vi "FP_Size to Largest Decoration.vi"(6 "Border Spacing (2 Px)":i32=2, 7 "Decoration index":i32, 8 "Error":errorcluster, 11 "VI Ref":refnum<vi>) -> (0 "Error Out":errorcluster, 2 "Front Panel.PanelBounds Out":T1, 3 "VI Ref Out":refnum<vi>)   [LabVIEW 2020]
doc: "Fits the vi's window to to the input GObject or largest decoration on the front panel"
uses:
  <vilib>/Utility/miscctls.llb/LVRectTypeDef.ctl
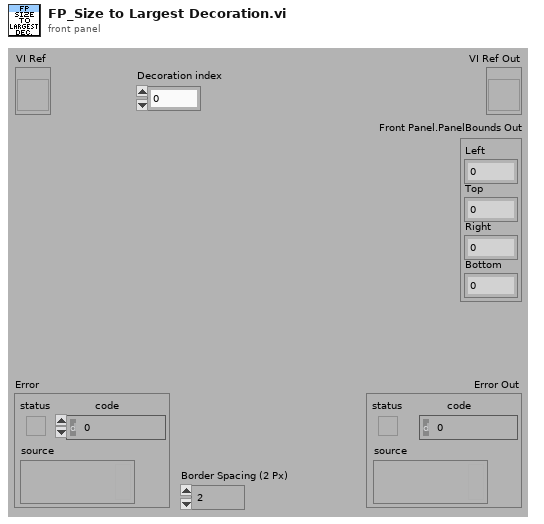
[diagram p1: front panel]
types:
  T1 = typedef "LVRectTypeDef.ctl" = cluster{"Left":i16, "Top":i16, "Right":i16, "Bottom":i16}
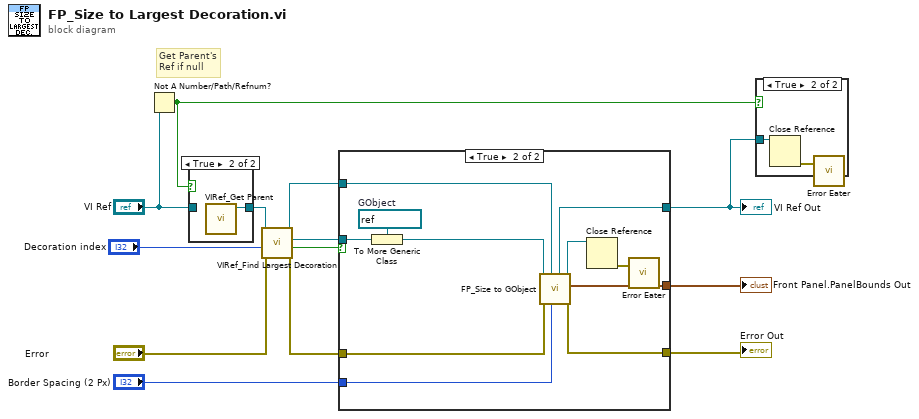
[diagram p0: block diagram]
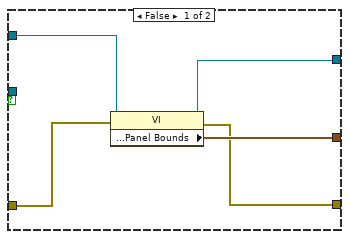
[diagram p2: hidden frame]
diagram:
  # "Get Parent's\nRef if null"
  n1 = Not A Number/Path/Refnum?(number/path/refnum="VI Ref") -> (NaN/Path/Refnum?=w12:bool)
  n2 = case shown="True" w12 {
    tunnel: [w14 w15] -> w6
    tunnel: "VI Ref" -> [w14 _]
    frame False {
    }
    frame True {
      n3 = call "VIRef_Get Parent.vi"() -> ("VI Refnum Out"=w15:refnum<vi>)  [unwired: 8 in, 3 out]
    }
  }
  n4 = call "VIRef_Find Largest Decoration.vi"("Error"="Error", "Decoration index"="Decoration index", "VI's Ref"=w6) -> ("Error Out"=w8:errorcluster, "Found"=w1:bool, "Decor Refnum Out"=w3:refnum<vi>, "Calling VI's Ref Out"=w7:refnum<vi>)  [unwired: 2 in, 3 out]
  n5 = case shown="True" w1 {
    tunnel: [w19 w31] -> w11
    tunnel: [w18 w30] -> w10
    tunnel: w8 -> [w17 w29]
    tunnel: w7 -> [w20 w28]
    tunnel: [w16 w27] -> w5
    tunnel: w3 -> [_ w26]
    tunnel: "Border Spacing (2 Px)" -> [_ w24]
    frame False {
      n6 = property on="Property Node" class="VI"(reference=w20, error in=w17) -> (reference out=w19:refnum<vi>, error out=w16:errorcluster, "Front Panel Window:Panel Bounds"=w18:T1)
    }
    frame True {
      w23 = refnum<vi> refnum  # GObject
      n7 = To More Generic Class(target class=w23, reference=w26) -> (generic class reference=w25:refnum<vi>)
      n8 = call "FP_Size to GObject.vi"("Border Spacing (2 Px)"=w24, "Calling VI's Ref"=w28, "Error"=w29, "GObj Refnum"=w25) -> ("Error Out"=w27:errorcluster, "Front Panel.PanelBounds Out"=w30:T1, "GObj Refnum Out"=w22:refnum<vi>, "Calling VI's Ref Out"=w31:refnum<vi>)  [unwired: 2 in, 2 out]
      n9 = Close Reference(reference=w22) -> (error out=w21:errorcluster)  [unwired: 1 in]
      n10 = call "Error Eater.vi"("error in (no error)"=w21) -> ()  [unwired: 2 in]
    }
  }
  "Error Out" <- w5
  "VI Ref Out" <- w11
  "Front Panel.PanelBounds Out" <- w10
  n11 = case shown="True" w12 {
    tunnel: w11 -> [_ w33]
    frame False {
    }
    frame True {
      n12 = Close Reference(reference=w33) -> (error out=w32:errorcluster)  [unwired: 1 in]
      n13 = call "Error Eater.vi"("error in (no error)"=w32) -> ()  [unwired: 2 in]
    }
  }
